vi "Play Speaker Sound.vi"(8 "error in (no error)":errorcluster, 11 "Frequencies IN":dbl[](array[numeric])=[233.04, 196.02, 233.04, 196.02, 233.04, 202.02, 240.02, 220.02, 262.0, 226.02, 269.03, 247.03, 277.03, 254.03, 285.04, 285.04, 302.07, 302.07, 320.05, 320.05, 349.08, 339.06, 370.09, 339.06, 415.01, 311.04, 427.05, 294.03, 466.08, 285.04, 494.07, 269.03, 508.16, 254.03, 571.17, 247.03, 587.19, 233.04, 604.14, 226.02, 640.11, 214.02, 659.21, 214.02, 679.1, 196.02, 698.17, 185.01, 719.21, 0.0, 740.18]) -> (0 "error out":errorcluster)   [LabVIEW 2017]
uses:
  <vilib>/sound2/lvsound2.llb/Sound Data Format.ctl
  <vilib>/sound2/lvsound2.llb/Sampling Mode.ctl
  <vilib>/sound2/lvsound2.llb/Sound Output Set Volume (Single).vi
  <vilib>/sound2/lvsound2.llb/Sound Output Write (DBL).vi
  <vilib>/Analysis/NI_AALBase.lvlib
panel:
  in  "sound format":T1={"sample rate (S/s)"=22050.0, "number of channels"=1, "bits per sample"=8}
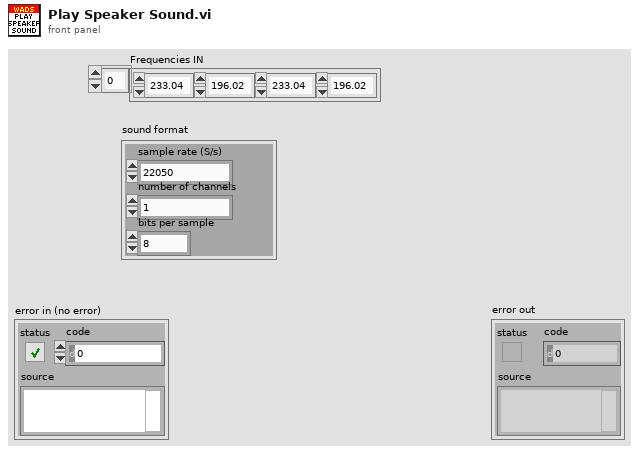
[diagram p1: front panel]
types:
  T1 = typedef "Sound Data Format.ctl" = cluster{"sample rate (S/s)":dbl, "number of channels":i32, "bits per sample":i32}
  T2 = typedef "Sampling Mode.ctl" = i32
  T3 = typedef "Sound Output Task ID.ctl" = u32
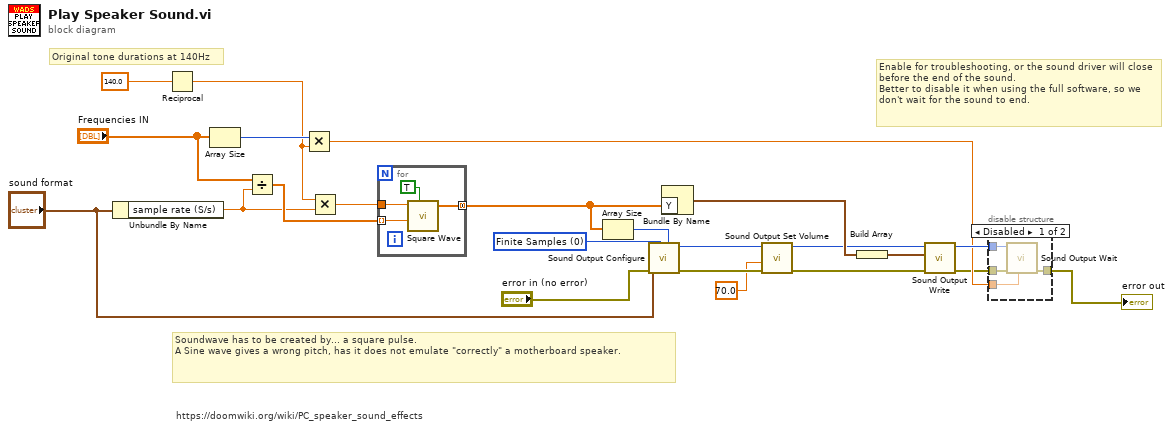
[diagram p0: block diagram]
diagram:
  w22 = T2 0 items=["Finite Samples", "Continuous Samples"] ("sample mode")
  # "Enable for troubleshooting, or the sound driver will close before the end of the sound.\nBetter to disable it when using the full software, so we don't wait for the sound to end."
  # "https://doomwiki.org/wiki/PC_speaker_sound_effects"
  # "Soundwave has to be created by... a square pulse.\nA Sine wave gives a wrong pitch, has it does not emulate \"correctly\" a motherboard speaker."
  # "Original tone durations at 140Hz"
  n1 = Unbundle By Name("sound format") -> ("sample rate (S/s)"=w11:dbl)
  n2 = Reciprocal(x=140.0 ("y")) -> (1/x=w10:dbl)
  n3 = Array Size(array="Frequencies IN") -> (size(s)=w21:i32)
  n4 = Divide(x="Frequencies IN", y=w11) -> (x/y=w16:dbl[])
  n5 = Multiply(x=w21, y=w10) -> (x*y=w13:dbl)
  n6 = Multiply(x=w10, y=w11) -> (x*y=w9:dbl)
  n7 = for {
    tunnel: [w24] -> w6 mode=concatenating
    tunnel: w9 -> [w26]
    tunnel: w16 -> [w25] mode=indexing
    n8 = call <vilib>:"Square Wave.vi"("samples"=w26, "reset phase"=TRUE, "frequency"=w25) -> ("square wave"=w24:dbl[])  [unwired: 3 in, 2 out]
  }
  n9 = Array Size(array=w6) -> (size(s)=w20:i32)
  n10 = call <vilib>:"Sound Output Configure.vi"("number of samples/ch"=w20, "sample mode"=w22, "error in (no error)"="error in (no error)", "sound format"="sound format") -> ("error out"=w4:errorcluster, "task ID"=w5:T3)  [unwired: 6 in]
  n11 = Bundle By Name("Y"=w6) -> (w19:waveform(dbl))  [unwired: 1 in]
  n12 = call-poly <vilib>:"Sound Output Set Volume.vi"("error in (no error)"=w4, "volume"=70.0, "task ID"=w5) -> ("error out"=w2:errorcluster, "task ID out"=w3:T3)  [unwired: 7 in]
  n13 = Build Array(w19) -> (w18:waveform(dbl)[])
  n14 = call-poly <vilib>:"Sound Output Write.vi"("error in (no error)"=w2, "data"=w18, "task ID"=w3) -> ("error out"=w8:errorcluster, "task ID out"=w14:T3)  [unwired: 7 in]
  n15 = disable-structure shown="Disabled" {
    disable-tunnel: w14 -> [w31 _]
    disable-tunnel: w13 -> [w30 _]
    disable-tunnel: w8 -> [w29 w32]
    disable-tunnel: [w28 w32] -> w7
    frame Disabled {
      n16 = call <vilib>:"Sound Output Wait.vi"("timeout (sec)"=w30, "error in (no error)"=w29, "task ID"=w31) -> ("error out"=w28:errorcluster)  [unwired: 7 in, 1 out]
    }
    frame Enabled {
    }
  }
  "error out" <- w7
